vi "Straightened Arcade.vi"(11 "Metrics In":T2={"Timestamp"=0, "Drive State"=enum."Initialize", "Throttle"=-0.0, "Turn"=0.0, "Heading"=0.0, "Absolute Heading"=0.0, "Left Velocity"=0.0, "Left Encoder"=0.0, "Right Velocity"=0.0, "Right Encoder"=0.0, "Left Power"=7.353305345843318, "Right Power"=-7.353305345843318, "Last Shift"=0, "Shift Started"=0, "Duration"=0}) -> (3 "Metrics Out":T2={"Timestamp"=0, "Drive State"=enum."Initialize", "Throttle"=-0.0, "Turn"=7.353785345866117, "Heading"=0.0, "Absolute Heading"=0.0, "Left Velocity"=0.0, "Left Encoder"=0.0, "Right Velocity"=0.0, "Right Encoder"=0.0, "Left Power"=7.353785345866117, "Right Power"=-7.353785345866117, "Last Shift"=0, "Shift Started"=0, "Duration"=0})   [LabVIEW 2014]
uses:
  Drive Metrics.ctl
  Drive States.ctl
  Support/LightningPID Settings.ctl
  Global Objects.vi
panel:
  in  "PID Settings":T1={"iMax"=0.1, "iMin"=-0.1, "iGain"=0.0, "pGain"=0.0, "dGain"=0.0, "MaxOutput"=1.0, "MinOutput"=-1.0, "AutoReset"=FALSE, "Tolerance"=2.0, "dSmoothing"=0.0}
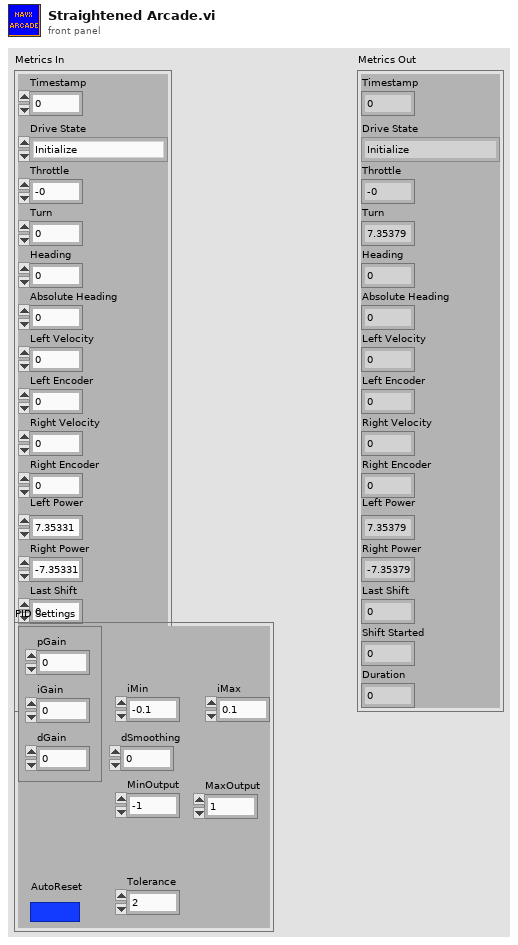
[diagram p1: front panel]
types:
  T1 = typedef "LightningPID Settings.ctl" = cluster{"iMax":dbl, "iMin":dbl, "iGain":dbl, "pGain":dbl, "dGain":dbl, "MaxOutput":dbl, "MinOutput":dbl, "AutoReset":bool, "Tolerance":dbl, "dSmoothing":dbl}
  T2 = typedef "Drive Metrics.ctl" = cluster{"Timestamp":u32, "Drive State":T3, "Throttle":dbl, "Turn":dbl, "Heading":dbl, "Absolute Heading":dbl, "Left Velocity":dbl, "Left Encoder":dbl, "Right Velocity":dbl, "Right Encoder":dbl, "Left Power":dbl, "Right Power":dbl, "Last Shift":u32, "Shift Started":u32, "Duration":u32}
  T3 = typedef "Drive States.ctl" = enum16{"Initialize", "Low Gear", "Up Shift Begin", "Up Shifting", "Up Shift Delay", "High Gear", "Down Shift Begin", "Down Shifting", "Down Shift Delay"}
  T4 = typedef "Configuration.ctl" = cluster{"Throttle Dead Zone":dbl, "Throttle Ramp Rate":dbl, "Turn Dead Zone":dbl, "Auton":cluster{"Motion Plan P":dbl, "Motion Plan I":dbl, "Motion Plan D":dbl}, "Auto Upshift Enabled":bool, "Upshift Min Throttle":dbl, "Upshift Min Velocity":dbl, "Min time before upshift":dbl, "Shift Throttle Detent":u32, "Min time before downshift":dbl, "Turn PID":cluster{"Motion Plan P":dbl, "Motion Plan I":dbl, "Motion Plan D":dbl}}
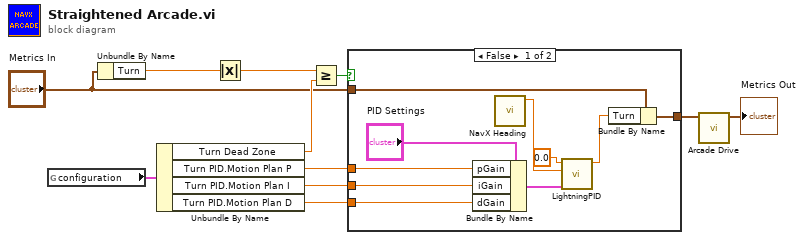
[diagram p0: block diagram]
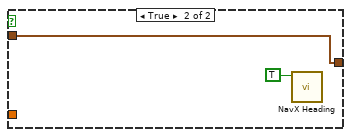
[diagram p2: hidden frame]
diagram:
  n1 = global read "Global Objects.vi" "configuration"() -> (w10:T4)
  n2 = Unbundle By Name("Metrics In") -> ("Turn"=w9:dbl)
  n3 = Unbundle By Name(w10) -> ("Turn Dead Zone"=w8:dbl, "Turn PID.Motion Plan P"=w4:dbl, "Turn PID.Motion Plan I"=w3:dbl, "Turn PID.Motion Plan D"=w2:dbl)
  n4 = Absolute Value(x=w9) -> (abs(x)=w1:dbl)
  n5 = Greater Or Equal?(x=w1, y=w8) -> (x >= y?=w7:bool)
  n6 = case shown="False" w7 {
    tunnel: [w20 w22] -> w6
    tunnel: "Metrics In" -> [w21 w22]
    tunnel: w4 -> [w19 _]
    tunnel: w3 -> [w18 _]
    tunnel: w2 -> [w17 _]
    frame False {
      n7 = Bundle By Name(cluster="PID Settings", "pGain"=w19, "iGain"=w18, "dGain"=w17) -> (w12:T1)
      n8 = call "NavX Heading.vi"() -> ("Heading"=w14:dbl)  [unwired: 9 in, 2 out]
      n9 = call "LightningPID.vi"("PID Settings"=w12, "Position"=w14, "Set Point"=0.0) -> ("Output"=w15:dbl)  [unwired: 8 in]
      n10 = Bundle By Name(cluster=w21, "Turn"=w15) -> (w20:T2)
    }
    frame True {
      n11 = call "NavX Heading.vi"("Zero Heading?"=TRUE) -> ()  [unwired: 8 in, 3 out]
    }
  }
  n12 = call "Arcade Drive.vi"("Metrics In"=w6) -> ("Metrics Out"=→"Metrics Out":T2)  [unwired: 6 in]
